vi "Alarm Temp.vi"(0 "Reference Cluster":T1, 1 "Temperatures":dbl[][](array[numeric])) -> ()   [LabVIEW 2017, in "GUI.lvlib"]
uses:
  GUI.lvlib
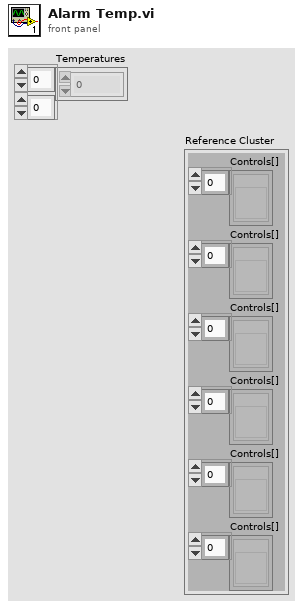
[diagram p1: front panel]
types:
  T1 = cluster{"Controls[]":refnum<vi>[], "Controls[]":refnum<vi>[], "Controls[]":refnum<vi>[], "Controls[]":refnum<vi>[], "Controls[]":refnum<vi>[], "Controls[]":refnum<vi>[]}
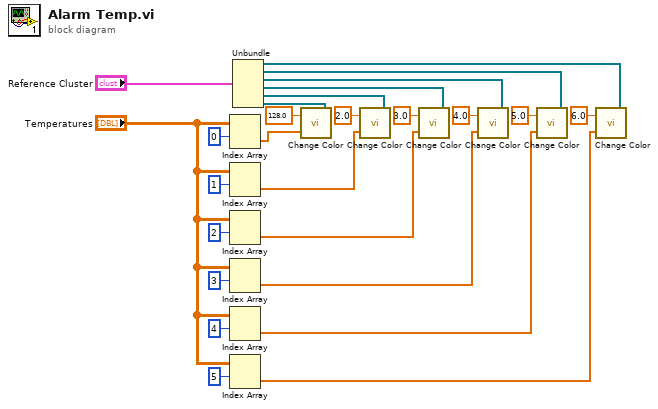
[diagram p0: block diagram]
diagram:
  n1 = Index Array(array="Temperatures", index (row)=0) -> (element=w6:dbl[])  [unwired: 1 in]
  n2 = Index Array(array="Temperatures", index (row)=1) -> (element=w5:dbl[])  [unwired: 1 in]
  n3 = Index Array(array="Temperatures", index (row)=2) -> (element=w4:dbl[])  [unwired: 1 in]
  n4 = Index Array(array="Temperatures", index (row)=3) -> (element=w3:dbl[])  [unwired: 1 in]
  n5 = Index Array(array="Temperatures", index (row)=4) -> (element=w2:dbl[])  [unwired: 1 in]
  n6 = Index Array(array="Temperatures", index (row)=5) -> (element=w1:dbl[])  [unwired: 1 in]
  n7 = Unbundle("Reference Cluster") -> ("Controls[]"=w24:refnum<vi>[], "Controls[]"=w23:refnum<vi>[], "Controls[]"=w22:refnum<vi>[], "Controls[]"=w21:refnum<vi>[], "Controls[]"=w20:refnum<vi>[], "Controls[]"=w19:refnum<vi>[])
  n8 = call "Change Color.vi"("Control References"=w19, "Temperatures"=w6, "Slave ID"=128.0) -> ()
  n9 = call "Change Color.vi"("Control References"=w20, "Temperatures"=w5, "Slave ID"=2.0) -> ()
  n10 = call "Change Color.vi"("Control References"=w21, "Temperatures"=w4, "Slave ID"=3.0) -> ()
  n11 = call "Change Color.vi"("Control References"=w22, "Temperatures"=w3, "Slave ID"=4.0) -> ()
  n12 = call "Change Color.vi"("Control References"=w23, "Temperatures"=w2, "Slave ID"=5.0) -> ()
  n13 = call "Change Color.vi"("Control References"=w24, "Temperatures"=w1, "Slave ID"=6.0) -> ()
